vi "test.vi"() -> ()   [LabVIEW 2011]
panel:
  out "result string":string
  out "string":string
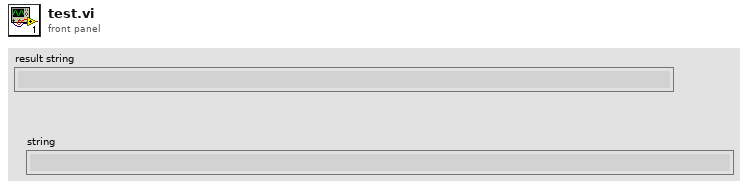
[diagram p1: front panel]
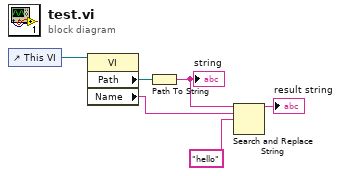
[diagram p0: block diagram]
diagram:
  n1 = control-ref of="This VI"() -> (w6:refnum<vi>)
  n2 = property class="VI"(reference=w6) -> ("Path"=w5:path, "Name"=w3:string)  [unwired: 1 in, 2 out]
  n3 = Path To String(path=w5) -> (string=w4:string)
  "string" <- w4
  n4 = Search and Replace String(input string=w4, search string=w3, replace string="hello" ("replace string (\"\")")) -> (result string=→"result string":string)  [unwired: 5 in, 3 out]
